vi "sub_pessimize_objective.vi"(8 "error in":errorcluster, 10 "Pessimize fun info":T1 {"Point selector"."Light number" min=0 max=5}, 11 "X":dbl[](array[numeric])) -> (0 "error out":errorcluster, 1 "f(X)":dbl, 2 "Error vector":dbl[](array[numeric]), 3 "Pose command":dbl[](array[numeric]))   [LabVIEW 2013]
uses:
  pessimize_objective_fun_info.ctl
  calibration/point_selector.ctl
  ui_override_opts.ctl
  <vilib>/Analysis/Matrix/Datatypes/RealMatrix.ctl
  <vilib>/Analysis/baseanly.llb/Real A x B.vi
  <vilib>/Analysis/NI_AALBase.lvlib
  <vilib>/Analysis/Matrix/NI_Matrix.lvlib
panel:
  # "This is the basic objective function for maximizing the ASAP error.  It finds the error at pose X with specified scaling and criterion."
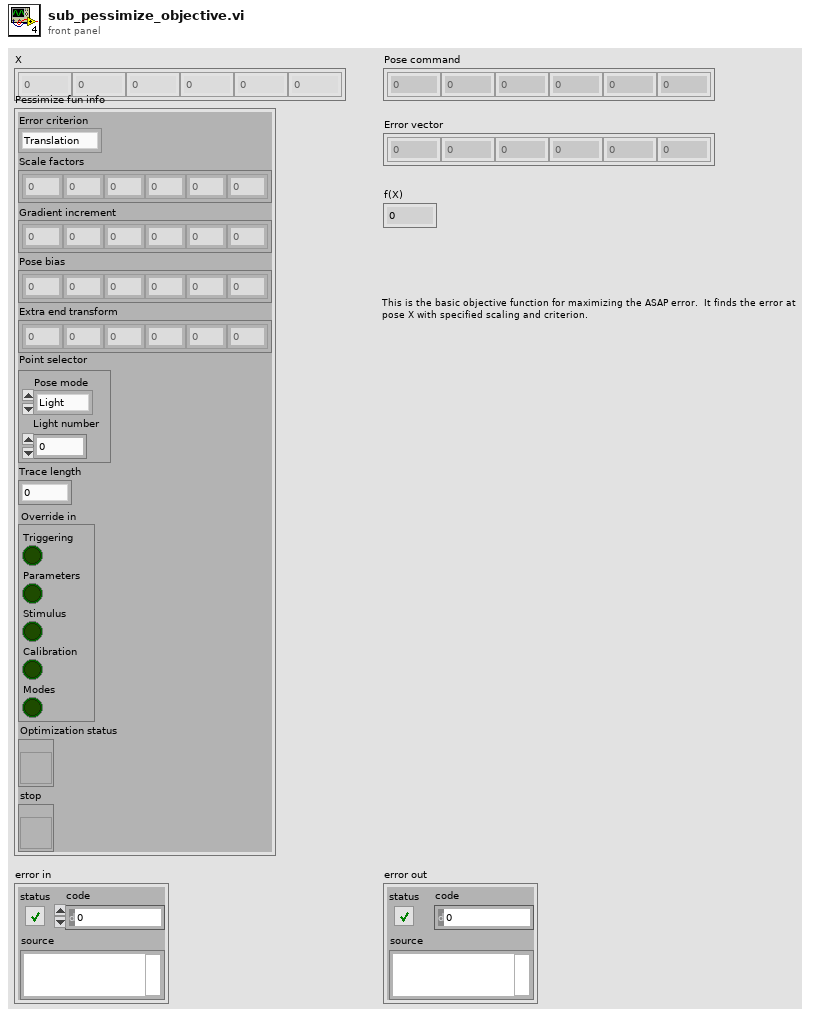
[diagram p1: front panel]
types:
  T1 = typedef "pessimize_objective_fun_info.ctl" = cluster{"Error criterion":enum16{"Translation", "Orientation", "Moment"}, "Scale factors":dbl[], "Gradient increment":dbl[], "Pose bias":dbl[], "Extra end transform":dbl[], "Point selector":T2, "Trace length":dbl, "Override in":T3, "Optimization status":refnum<vi>, "stop":refnum<vi>}
  T2 = typedef "point_selector.ctl" = cluster{"Pose mode":enum16{"Light", "Handle", "Output"}, "Light number":i32}
  T3 = typedef "ui_override_opts.ctl" = cluster{"Triggering":bool, "Parameters":bool, "Stimulus":bool, "Calibration":bool, "Modes":bool}
  T4 = typedef "NI_Matrix.lvlib/RealMatrix.ctl" = dbl[][]
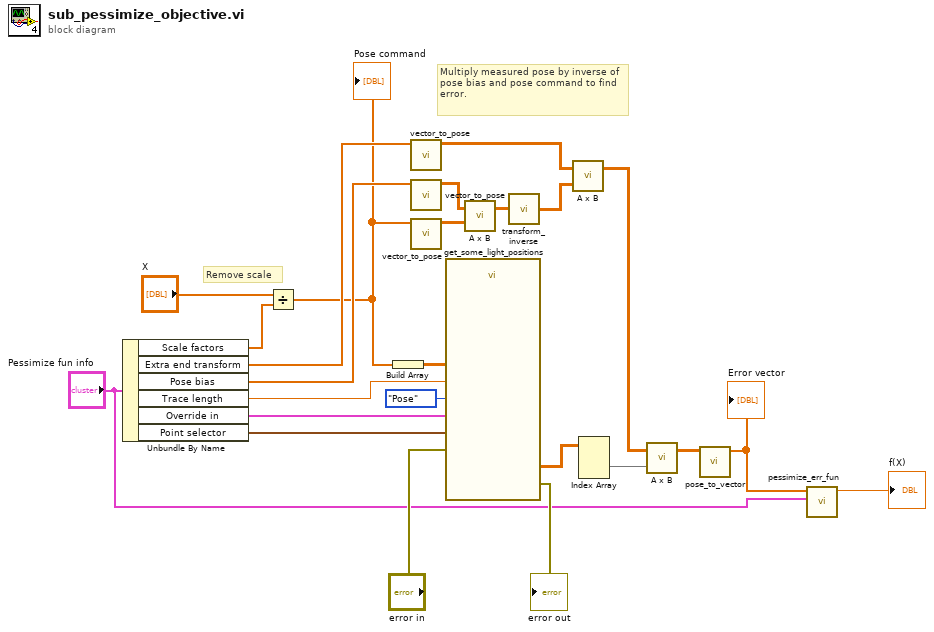
[diagram p0: block diagram]
diagram:
  # "Multiply measured pose by inverse of pose bias and pose command to find error."
  # "Remove scale"
  n1 = Unbundle By Name("Pessimize fun info") -> ("Scale factors"=w11:dbl[], "Extra end transform"=w6:dbl[], "Pose bias"=w10:dbl[], "Trace length"=w22:dbl, "Override in"=w14:T3, "Point selector"=w15:T2)
  n2 = Divide(x="X", y=w11) -> (x/y=w1:dbl[])
  "Pose command" <- w1
  n3 = Build Array(w1) -> (w13:dbl[][])
  n4 = call "vector_to_pose.vi"("Pose vector"=w6) -> ("Pose"=w5:T4)  [unwired: 10 in]
  n5 = call "vector_to_pose.vi"("Pose vector"=w10) -> ("Pose"=w8:T4)  [unwired: 10 in]
  n6 = call "vector_to_pose.vi"("Pose vector"=w1) -> ("Pose"=w7:T4)  [unwired: 10 in]
  n7 = call "get_some_light_positions.vi"("Trace length"=w22, "Point selector"=w15, "Position mode"=enum16{"Absolute axis", "Relative axis", "Pose"}."Pose", "error in"="error in", "Sequence"=w13, "Override"=w14) -> ("error out"=→"error out":errorcluster, "Poses"=w17:dbl[][][])  [unwired: 3 in, 1 out]
  n8 = call-poly <vilib>:"A x B.vi"("B"=w7, "A"=w8) -> ("A x B"=w9:T4)  [unwired: 1 out]
  n9 = call "transform_inverse.vi"("Transform"=w9) -> ("Inverse transform"=w4:T4)
  n10 = call-poly <vilib>:"A x B.vi"("B"=w4, "A"=w5) -> ("A x B"=w2:T4)  [unwired: 1 out]
  n11 = Index Array(array=w17) -> (element=w3:dbl[][])  [unwired: 3 in]
  n12 = call-poly <vilib>:"A x B.vi"("B"=w3, "A"=w2) -> ("A x B"=w18:T4)  [unwired: 1 out]
  n13 = call "pose_to_vector.vi"("Pose"=w18) -> ("Pose vector"=w21:dbl[])  [unwired: 10 in]
  "Error vector" <- w21
  n14 = call "pessimize_err_fun.vi"("Pessimize fun info"="Pessimize fun info", "Error"=w21) -> ("Result"=→"f(X)":dbl)  [unwired: 9 in]
